vi "Generate missing timelapse header file.vi"(8 "error in (no error)":errorcluster, 11 "Timelapse data folder path":path) -> ()   [LabVIEW 2013]
uses:
  Functional Imaging Viewer/SubVIs/Experiment header interface/Typedefs/Header file type enum.ctl
  Functional Imaging Viewer/SubVIs/Experiment header interface/Typedefs/Header file interface module functions enum.ctl
  Globals/gl_Time series viewer globals.vi
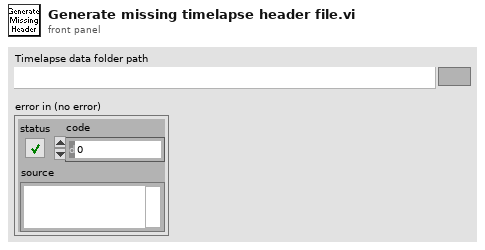
[diagram p1: front panel]
types:
  T1 = typedef "Header file interface module functions enum.ctl" = enum16{"Load experiment header file", "Save experiment header file", "Clear stored values", "Read stored values", "Update specific value in memory", "Update all values in memory"}
  T2 = typedef "Header file type enum.ctl" = enum16{"All parameters", "Params for funct acq w ROI or mscn", "Params for funct acq w rectangles", "Live imaging header parameters", "AOL Parameters"}
  T3 = typedef "AVI playback header info cluster.ctl" = cluster{"Frame Size":u32, "AOD fill time (us)":dbl, "Dwell time (us)":dbl, "Frame period (ms)":dbl, "Number of Miniscans":u16, "Number of Pixels in Miniscan":u16}
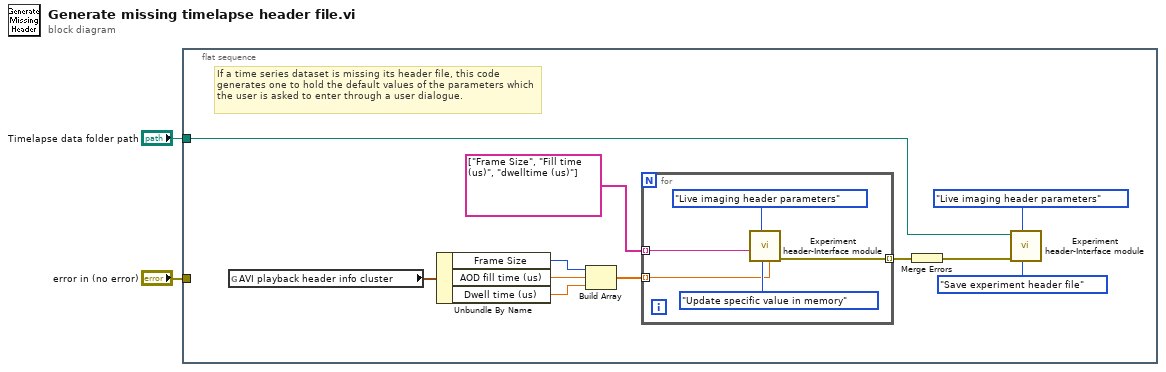
[diagram p0: block diagram]
diagram:
  n1 = flat-sequence {
    tunnel: "error in (no error)" -> [_]
    tunnel: "Timelapse data folder path" -> [w10]
    frame #0 {
      # "If a time series dataset is missing its header file, this code generates one to hold the default values of the parameters which the user is asked to enter through a user dialogue."
      n2 = global read "gl_Time series viewer globals.vi" "AVI playback header info cluster"() -> (w11:T3)
      n3 = Unbundle By Name(w11) -> ("Frame Size"=w9:u32, "AOD fill time (us)"=w8:dbl, "Dwell time (us)"=w7:dbl)
      n4 = Build Array(w9, w8, w7) -> (w6:dbl[])
      n5 = for {
        tunnel: w6 -> [w16] mode=indexing
        tunnel: string[] ["Frame Size", "Fill time (us)", "dwelltime (us)"] -> [w15] mode=indexing
        tunnel: [w14] -> w4 mode=indexing
        n6 = call "Experiment header-Interface module.vi"("New Value"=w16, "Name of parameter to update"=w15, "Header file type"=Header_file_type_enum."Live imaging header parameters", "Function"=Header_file_interface_module_functions_enum."Update specific value in memory") -> ("error out"=w14:errorcluster)  [unwired: 6 in, 1 out]
      }
      n7 = Merge Errors(w4) -> (w3:errorcluster)
      n8 = call "Experiment header-Interface module.vi"("Header file type"=Header_file_type_enum."Live imaging header parameters", "error in (no error)"=w3, "Function"=Header_file_interface_module_functions_enum."Save experiment header file", "Experiment data folder path"=w10) -> ()  [unwired: 6 in, 2 out]
    }
  }
